vi "update channel selections.vi"(8 "data":T1, 11 "channelSelection":u16) -> (0 "data out":T1, 3 "selected channel":string)   [LabVIEW 2018]
uses:
  liveData cluster.ctl
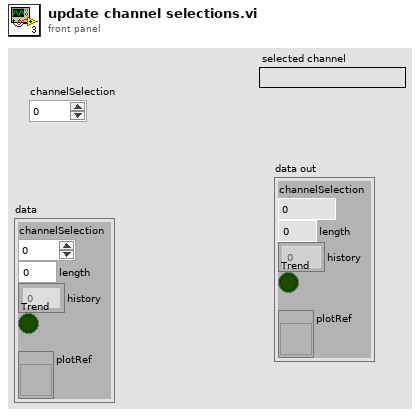
[diagram p1: front panel]
types:
  T1 = typedef "liveData cluster.ctl" = cluster{"channelSelection":i32, "length":dbl, "history":dbl[], "Trend":bool, "plotRef":refnum<vi>}
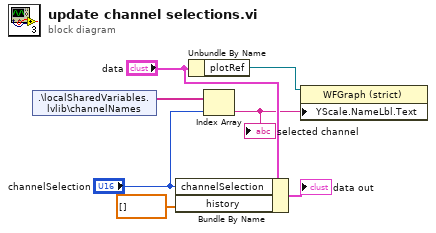
[diagram p0: block diagram]
diagram:
  n1 = shared-variable ".\\localSharedVariables.lvlib\\channelNames"() -> (w6:string[])  [unwired: 1 in, 1 out]
  n2 = Bundle By Name(cluster="data", "channelSelection"="channelSelection", "history"=dbl[] []) -> (→"data out":T1)
  n3 = Unbundle By Name("data") -> ("plotRef"=w4:refnum<vi>)
  n4 = Index Array(array=w6, index="channelSelection") -> (element=w3:string)
  "selected channel" <- w3
  n5 = property class="WFGraph (strict)"(reference=w4, "YScale.NameLbl.Text"=w3) -> ()  [unwired: 1 in, 2 out]
